vi "NumSteps.vi"(9 "Step":dbl, 10 "Stop":dbl, 11 "Start":dbl) -> (3 "Numeric":dbl)   [LabVIEW 2018]
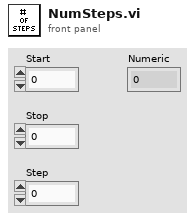
[diagram p1: front panel]
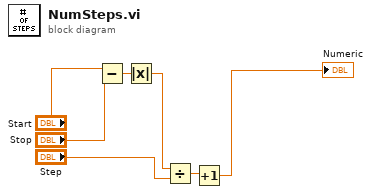
[diagram p0: block diagram]
diagram:
  n1 = Subtract(x="Start", y="Stop") -> (x-y=w5:dbl)
  n2 = Absolute Value(x=w5) -> (abs(x)=w6:dbl)
  n3 = Divide(x=w6, y="Step") -> (x/y=w2:dbl)
  n4 = Increment(x=w2) -> (x+1=→"Numeric":dbl)
